vi "Configure Dialog.vi"(8 "error in (no error)":errorcluster, 11 "Configure TrigLevel Msg.lvclass":refnum<class "Configure TrigLevel Msg.lvclass">) -> (0 "error out":errorcluster, 2 "Ok?":bool, 3 "Configure TrigLevel Msg.lvclass":refnum<class "Configure TrigLevel Msg.lvclass">)   [LabVIEW 2015, in "CS++MCS.lvlib" / "Configure TrigLevel Msg.lvclass"]
uses:
  Configure TrigLevel Msg.lvclass
  Configure TrigLevel Msg.lvclass/Configure TrigLevel Msg.ctl
panel:
  in  "TrigLvl":dbl[unit]
  in  "Cancel Button":bool
  in  "OK Button":bool
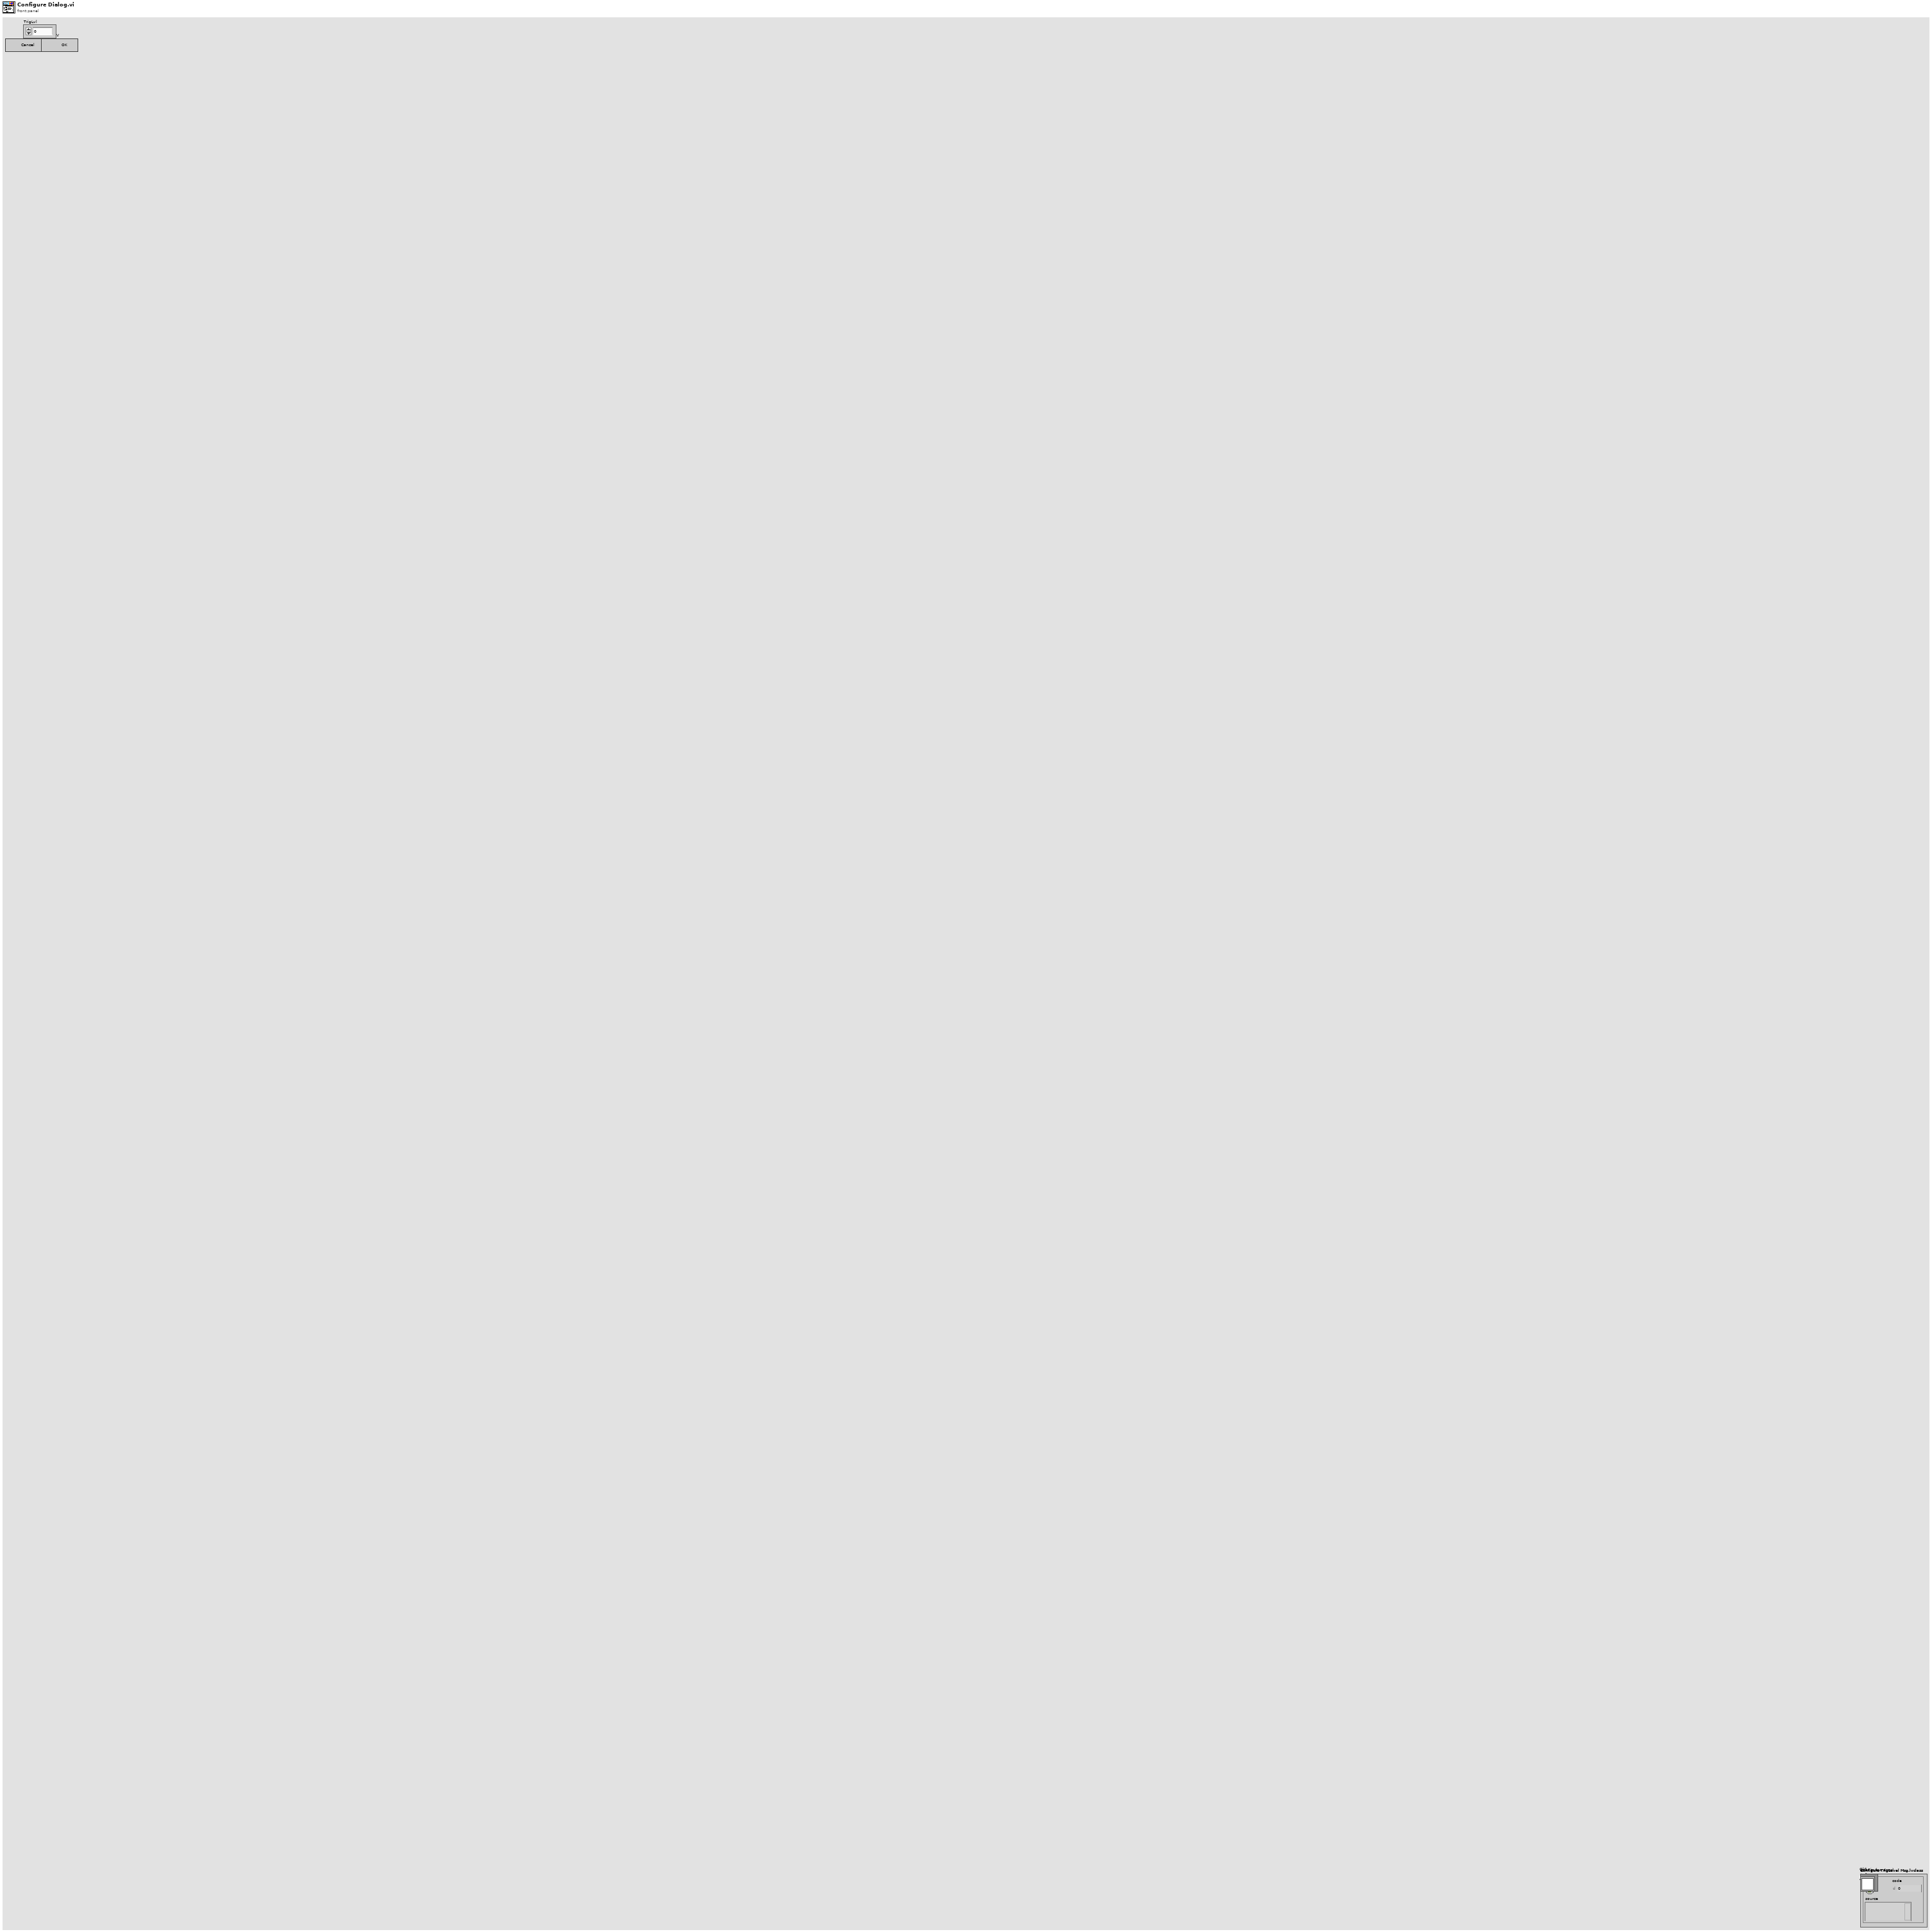
[diagram p1: front panel]
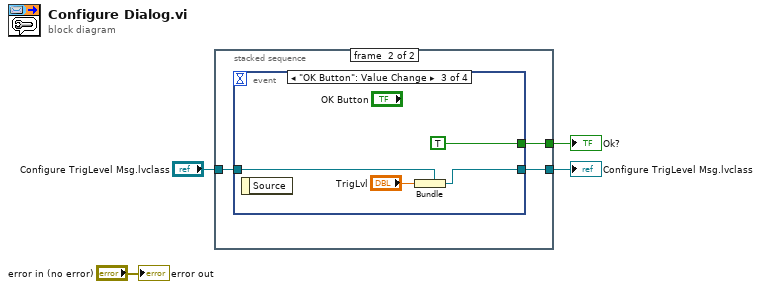
[diagram p0: block diagram]
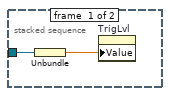
[diagram p2: hidden frame]
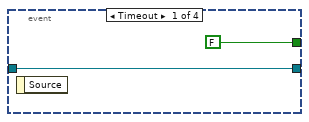
[diagram p3: hidden frame]
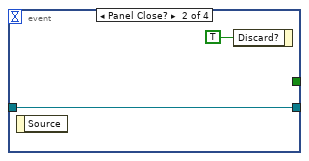
[diagram p4: hidden frame]
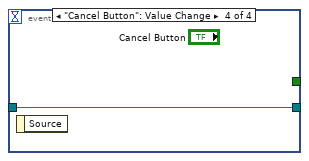
[diagram p5: hidden frame]
diagram:
  n1 = stacked-sequence {
    tunnel: [_ w9] -> w3
    tunnel: [_ w8] -> w2
    tunnel: "Configure TrigLevel Msg.lvclass" -> [w6 w7]
    frame #0 {
      n2 = Unbundle ("Seq0Unbundler")(w6) -> (w5:dbl[unit])
      n3 = property on="TrigLvl" class="DigNum (strict)"("Value"=w5) -> ()  [unwired: 2 in, 2 out]
    }
    frame #1 {
      n4 = event shown="[2] \"OK Button\": Value Change" {
        selector: _ -> [_ _ _ _]
        dyn-events: _ -> [_ _ _ _]
        timeout: _ -> [_ _ _ _]
        tunnel: [w10 w12 w15 w18] -> w8
        tunnel: w7 -> [w10 w12 w17 w18]
        tunnel: [FALSE _ TRUE _] -> w9
        event Timeout {
          n5 = event-data() -> ()  [unwired: 1 in, 1 out]
        }
        event Panel Close? {
          n6 = event-data() -> ()  [unwired: 1 in, 1 out]
          n7 = event-data ("Event Filter Node")("Discard?"=TRUE) -> ()  [unwired: 1 in, 1 out]
        }
        event "OK Button": Value Change {
          n8 = event-data() -> ()  [unwired: 1 in, 1 out]
          n9 = Bundle ("Main-Bundler")(cluster=w17, "TrigLvl") -> (w15:refnum<class "Configure TrigLevel Msg.lvclass">)
        }
        event "Cancel Button": Value Change {
          n10 = event-data() -> ()  [unwired: 1 in, 1 out]
        }
      }
    }
  }
  "Ok?" <- w3
  "Configure TrigLevel Msg.lvclass" <- w2
  "error out" <- "error in (no error)"
